vi "Error to String.vi"(6 "Error Array":errorcluster[](array[cluster]), 7 "Error In":errorcluster) -> (1 "Error String":string, 3 "error status":bool)   [LabVIEW 2011]
doc: "Converts error message(s) to a string. Can accept a single error message, an array of error messages, or both. Unlike the 'Merge Errors.vi', this VI actually combines ALL of the errors that occured into one long string.\n\nError in - Single error message cluster in\nError Array - Array of error message clusters in\n\nStatus - Indicates error status. True indicates error has occured.\nError String - A string of all the error codes, conditions, and messages concatenated into one long string."
uses:
  <vilib>/Utility/error.llb/DialogType.ctl
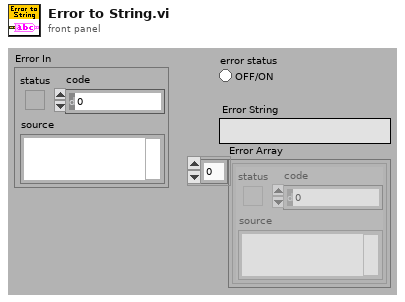
[diagram p1: front panel]
types:
  T1 = typedef "DialogType.ctl" = u16
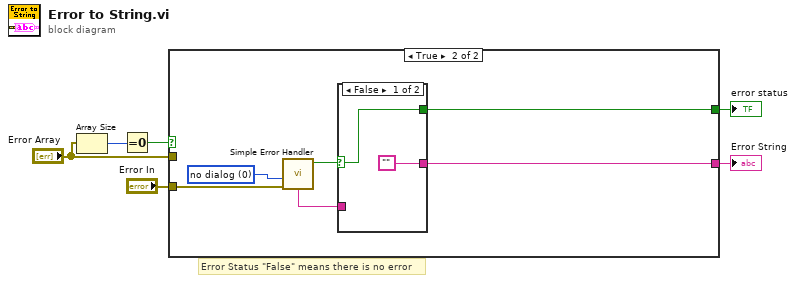
[diagram p0: block diagram]
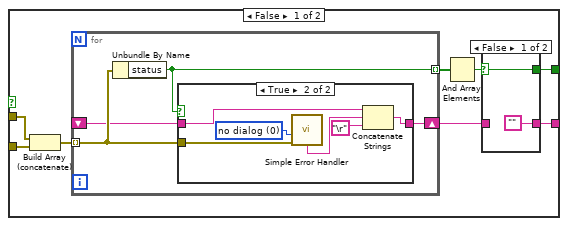
[diagram p2: hidden frame]
diagram:
  # "Error Status \"False\" means there is no error"
  n1 = Array Size(array="Error Array") -> (size(s)=w3:i32)
  n2 = Equal To 0?(x=w3) -> (x = 0?=w2:bool)
  n3 = case shown="True" w2 {
    tunnel: "Error In" -> [w11 w34]
    tunnel: [w7 w32] -> w5
    tunnel: [w9 w33] -> w4
    tunnel: "Error Array" -> [w12 _]
    frame False {
      n4 = Build Array (concatenate)(w12, w11) -> (w14:errorcluster[])
      n5 = for {
        tunnel: w14 -> [w22] mode=indexing
        shift-right: [w21] -> w8
        shift-left: _ -> [w20]
        tunnel: [w19] -> w13 mode=indexing
        n6 = Unbundle By Name(w22) -> ("status"=w19:bool)
        n7 = case shown="True" w19 {
          tunnel: w22 -> [_ w29]
          tunnel: [w23 w27] -> w21
          tunnel: w20 -> [w23 w28]
          frame False {
          }
          frame True {
            w24 = T1 0 items=["no dialog", "OK message", "continue or stop message", "OK message + warnings", "continue/stop + warnings"] ("type of dialog (OK msg:1)")
            n8 = call <vilib>:"Simple Error Handler.vi"("type of dialog (OK msg:1)"=w24, "error in (no error)"=w29) -> ("message"=w26:string)  [unwired: 3 in, 4 out]
            n9 = Concatenate Strings(w28, w26, "\r") -> (w27:string)
          }
        }
      }
      n10 = And Array Elements(Boolean array=w13) -> (logical AND=w10:bool)
      n11 = case shown="False" w10 {
        selector: w10 -> [w16 w17]
        tunnel: ["" w18] -> w9
        tunnel: w8 -> [_ w18]
        tunnel: [w16 w17] -> w7
        frame False {
        }
        frame True {
        }
      }
    }
    frame True {
      w35 = T1 0 items=["no dialog", "OK message", "continue or stop message", "OK message + warnings", "continue/stop + warnings"] ("type of dialog (OK msg:1)")
      n12 = call <vilib>:"Simple Error Handler.vi"("type of dialog (OK msg:1)"=w35, "error in (no error)"=w34) -> ("error?"=w30:bool, "message"=w31:string)  [unwired: 3 in, 3 out]
      n13 = case shown="False" w30 {
        selector: w30 -> [w37 w38]
        tunnel: ["" w39] -> w33
        tunnel: w31 -> [_ w39]
        tunnel: [w37 w38] -> w32
        frame False {
        }
        frame True {
        }
      }
    }
  }
  "error status" <- w5
  "Error String" <- w4
